vi "Sequence-StepFollw.vi"(8 "error in (no error)":errorcluster, 10 "Row Index":i32, 11 "MCListbox Refnum":refnum<vi>) -> (0 "error out":errorcluster, 3 "MCListbox Refnum(dup)":refnum<vi>)   [LabVIEW 2020, in "CSMScript-Engine(Lite).lvlib"]
uses:
  CSMScript-Engine(Lite).lvlib
  <vilib>/Utility/miscctls.llb/LVRowAndColumnUnsignedTypeDef.ctl
panel:
  # "Connector Pane"
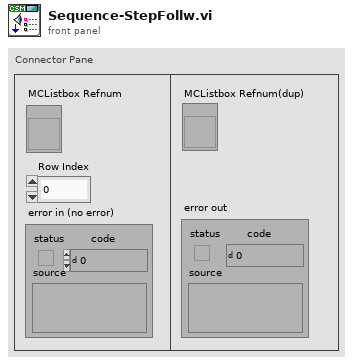
[diagram p1: front panel]
types:
  T1 = typedef "LVRowAndColumnUnsignedTypeDef.ctl" = cluster{"Row":u32, "Column":u32}
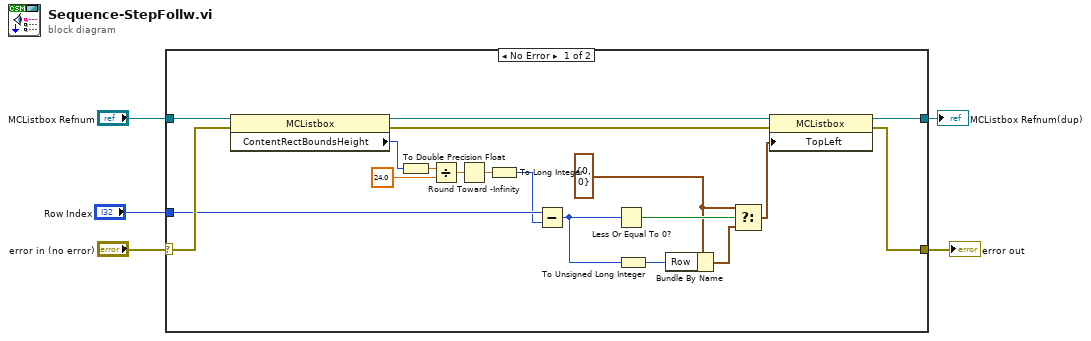
[diagram p0: block diagram]
diagram:
  n1 = case shown="No Error" "error in (no error)" {
    selector: "error in (no error)" -> [w23 w26]
    tunnel: [w6 w26] -> w5
    tunnel: "MCListbox Refnum" -> [w24 w25]
    tunnel: [w7 w25] -> w2
    tunnel: "Row Index" -> [w16 _]
    frame No Error {
      w12 = T1 {"Row"=0, "Column"=0} ("Top Left Visible Cell")
      n2 = property class="MCListbox"(reference=w24, error in=w23) -> (reference out=w10:refnum<vi>, error out=w9:errorcluster, "ContentRectBoundsHeight"=w21:i32)
      n3 = To Double Precision Float(number=w21) -> (double precision float=w20:dbl)
      n4 = Divide(x=w20, y=24.0) -> (x/y=w14:dbl)
      n5 = Round Toward -Infinity(1:w14) -> (0:w15:dbl)
      n6 = To Long Integer(number=w15) -> (32bit integer=w13:i32)
      n7 = Subtract(x=w16, y=w13) -> (x-y=w17:i32)
      n8 = Less Or Equal To 0?(x=w17) -> (x <= 0?=w19:bool)
      n9 = To Unsigned Long Integer(number=w17) -> (unsigned 32bit integer=w11:u32)
      n10 = Bundle By Name(cluster=w12, "Row"=w11) -> (w18:T1)
      n11 = Select(t=w12, s=w19, f=w18) -> (s? t:f=w8:T1)
      n12 = property class="MCListbox"(reference=w10, error in=w9, "TopLeft"=w8) -> (reference out=w7:refnum<vi>, error out=w6:errorcluster)
    }
    frame Error {
    }
  }
  "error out" <- w5
  "MCListbox Refnum(dup)" <- w2
